vi "readFromTXTForXMLFiles.vi"(0 "input_path_dataSource":path, 5 "input_array_startTime":string[](array[string])=["1", "2"], 9 "input_array_endTime":string[](array[string])=["2", "3"]) -> (1 "paddle_TDD22":string[](array[string]), 2 "show_Terminal Point":dbl[](array[numeric]), 3 "show_array_TDD11":string[](array[string]), 4 "show_array_SDD21":string[](array[string]), 6 "show_array_SDD11_Max":string[](array[string]), 8 "show_array_ILD_Max":string[](array[string]), 10 "show_array_SCC11_Max":string[](array[string]), 11 "paddle_TDD11":string[](array[string]), 12 "show_array_Next":string[](array[string]), 13 "show_Cable Point":dbl[](array[numeric]), 14 "show_array_TDD22":string[](array[string]))   [LabVIEW 2011]
uses:
  <vilib>/Utility/file.llb/Read From Spreadsheet File (string).vi
panel:
  out "子数组":string[](array[string])
  out "show_array_index":dbl[](array[numeric])
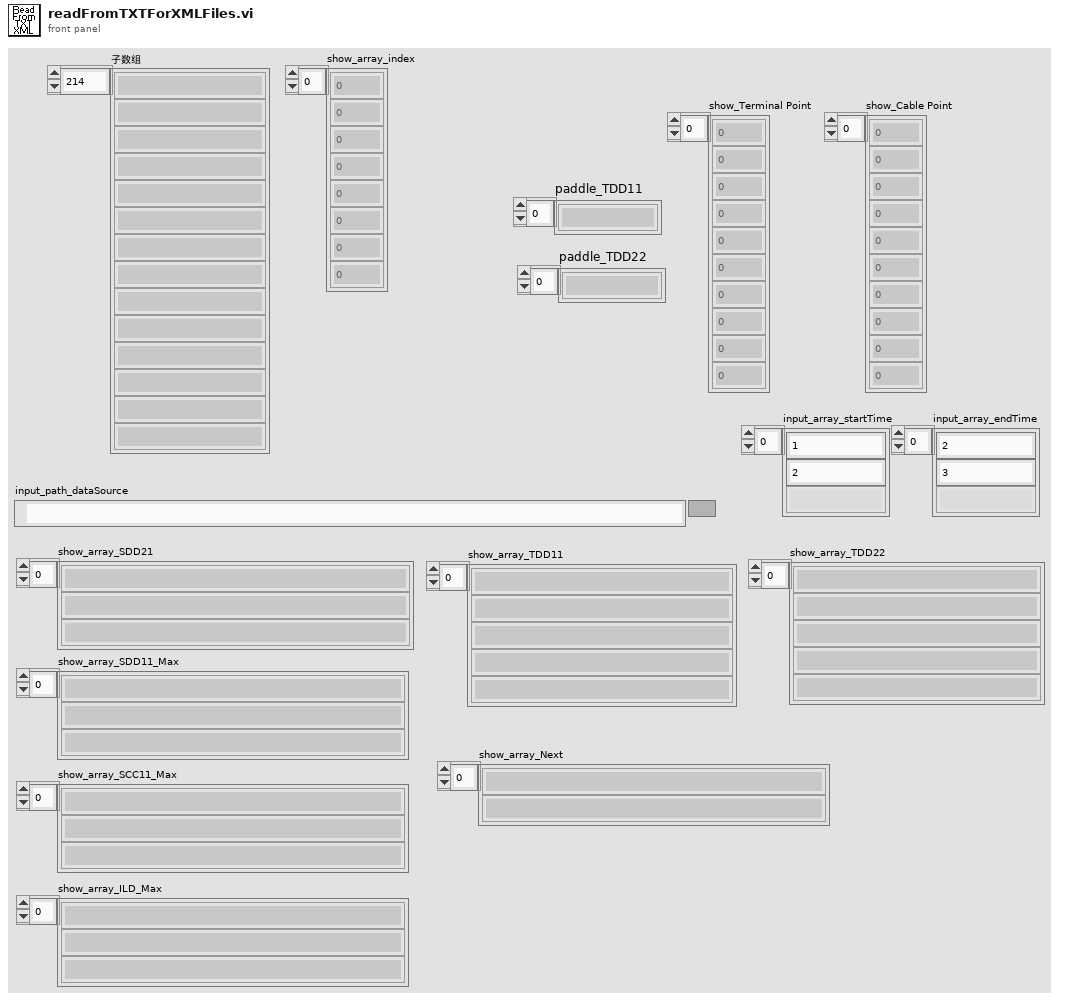
[diagram p1: front panel]
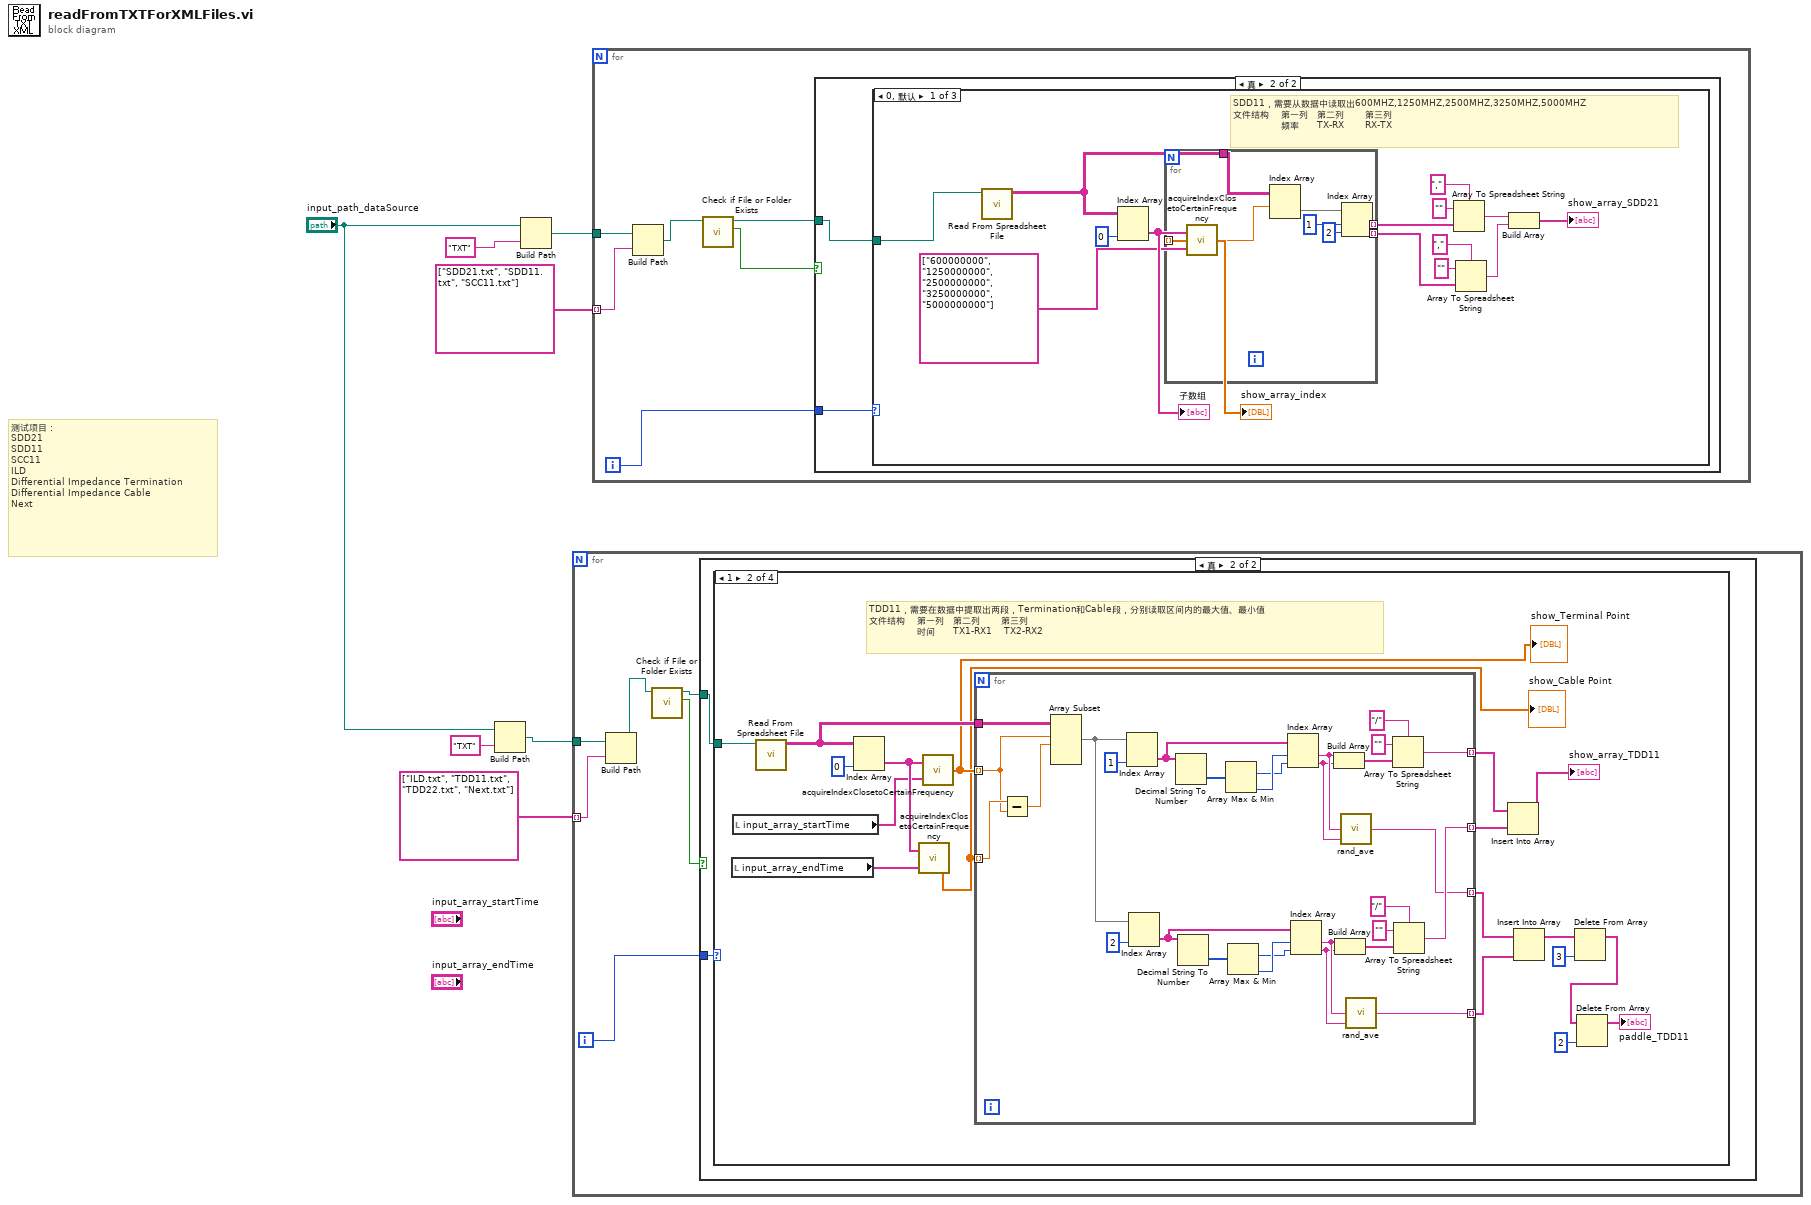
[diagram p0: block diagram]
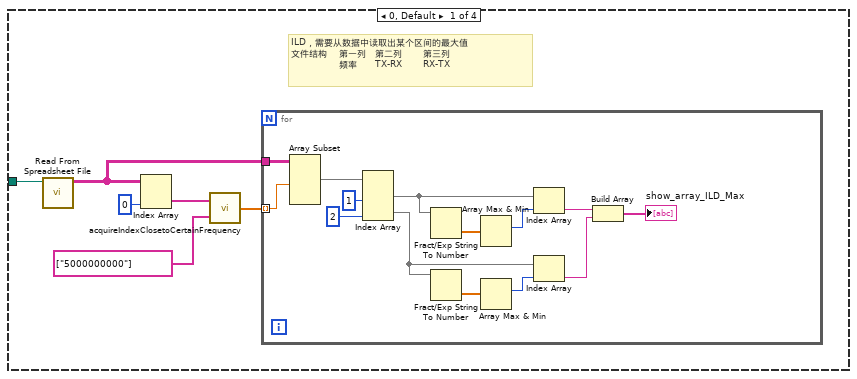
[diagram p3: hidden frame]
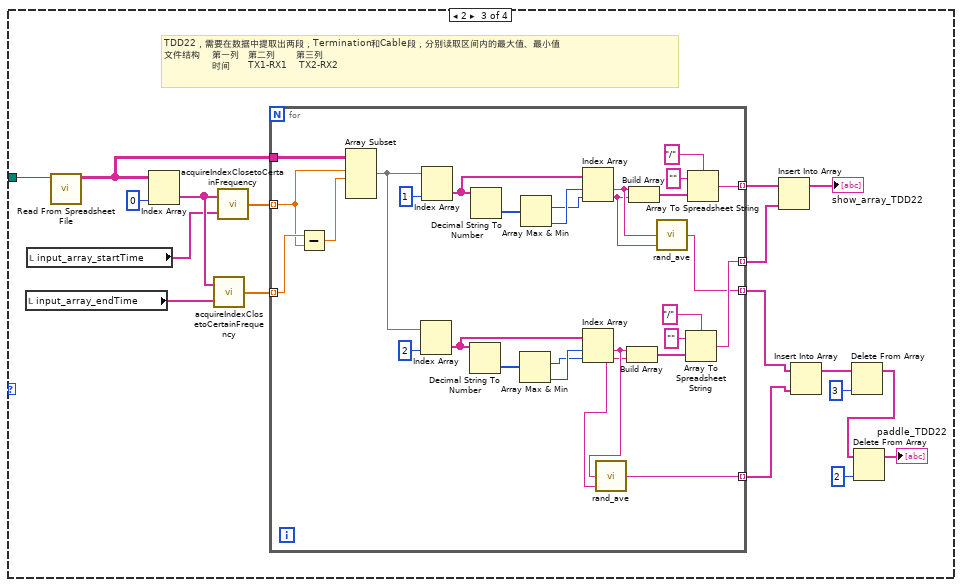
[diagram p4: hidden frame]
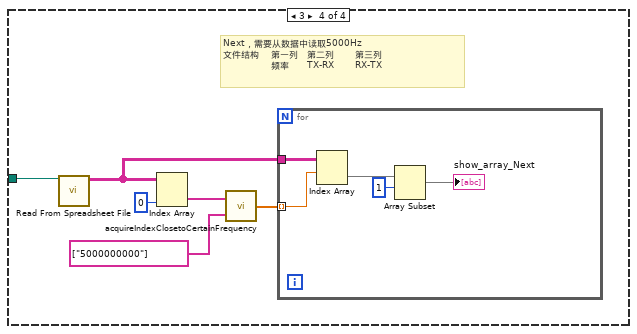
[diagram p5: hidden frame]
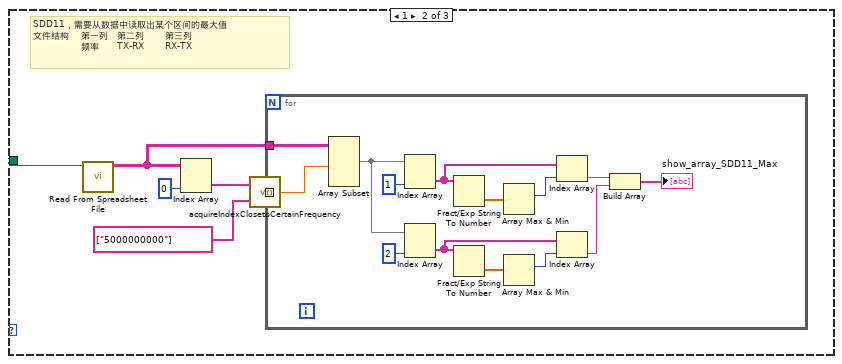
[diagram p7: hidden frame]
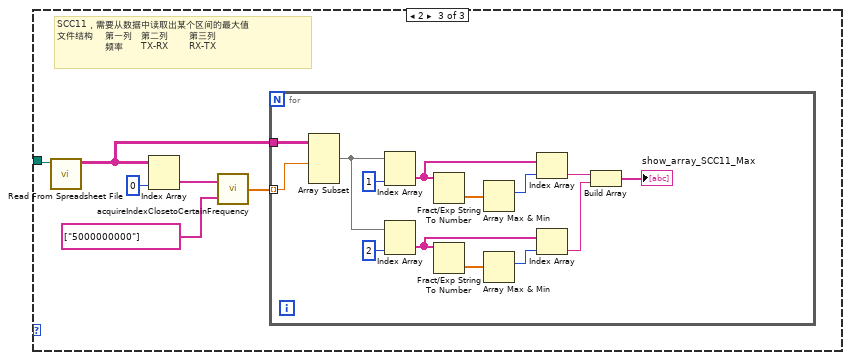
[diagram p8: hidden frame]
diagram:
  # "测试项目：\nSDD21\nSDD11\nSCC11\nILD\nDifferential Impedance Termination\nDifferential Impedance Cable\nNext"
  n1 = Build Path(base path="input_path_dataSource", name or relative path="TXT" ("名称或相对路径")) -> (appended path=w1:path)
  n2 = Build Path(base path="input_path_dataSource", name or relative path="TXT" ("名称或相对路径")) -> (appended path=w4:path)
  n3 = for {
    tunnel: string[] ["ILD.txt", "TDD11.txt", "TDD22.txt", "Next.txt"] -> [w12] mode=indexing
    tunnel: w1 -> [w13]
    i -> [w11]
    n4 = Build Path(base path=w13, name or relative path=w12) -> (appended path=w10:path)
    n5 = call <vilib>:"Check if File or Folder Exists.vi"("path"=w10) -> ("file or folder exists?"=w9:bool, "dup path"=w8:path)  [unwired: 8 in, 1 out]
    n6 = case shown="真" w9 {
      tunnel: w11 -> [_ w15]
      tunnel: w8 -> [_ w14]
      frame False {
      }
      frame True {
        n7 = case shown="1" w15 {
          tunnel: w14 -> [w21 w36 w97 w130]
          frame 0, Default {
            # "ILD，需要从数据中读取出某个区间的最大值\n文件结构    第一列   第二列       第三列       \n                频率      TX-RX       RX-TX"
            n8 = call-poly <vilib>:"Read From Spreadsheet File.vi"("file path (dialog if empty)"=w21) -> ("all rows"=w17:string[][])  [unwired: 6 in, 4 out]
            n9 = Index Array(array=w17, index (col)=0 ("禁用的索引 (列)")) -> (element=w19:string[])  [unwired: 1 in]
            n10 = call "acquireIndexClosetoCertainFrequency.vi"("input_array_freDemand"=string[] ["5000000000"], "input_array_freArray"=w19) -> ("show_array_index"=w16:dbl[])
            n11 = for {
              tunnel: w17 -> [w35]
              tunnel: w16 -> [w34] mode=indexing
              n12 = Array Subset(array=w35, length (row)=w34) -> (w33:string[][])  [unwired: 3 in]
              n13 = Index Array(array=w33, index (col) #1=1 ("禁用的索引 (列)"), index (col) #2=2 ("索引 (列)")) -> (element #1=w26:string[], element #2=w25:string[])  [unwired: 2 in]
              n14 = Fract/Exp String To Number(string=w26) -> (number=w30:dbl[])  [unwired: 3 in, 1 out]
              n15 = Fract/Exp String To Number(string=w25) -> (number=w29:dbl[])  [unwired: 3 in, 1 out]
              n16 = Array Max & Min(array=w30) -> (max index (indices)=w28:i32)  [unwired: 3 out]
              n17 = Array Max & Min(array=w29) -> (max index (indices)=w27:i32)  [unwired: 3 out]
              n18 = Index Array(array=w26, index=w28) -> (element=w23:string)
              n19 = Index Array(array=w25, index=w27) -> (element=w22:string)
              n20 = Build Array(w23, w22) -> (→"show_array_ILD_Max":string[])
            }
          }
          frame 1 {
            # "TDD11，需要在数据中提取出两段，Termination和Cable段，分别读取区间内的最大值、最小值\n文件结构    第一列   第二列       第三列\n                时间      TX1-RX1    TX2-RX2"
            n21 = local read "input_array_endTime"() -> (w45:string[])
            n22 = local read "input_array_startTime"() -> (w44:string[])
            n23 = call-poly <vilib>:"Read From Spreadsheet File.vi"("file path (dialog if empty)"=w36) -> ("all rows"=w52:string[][])  [unwired: 6 in, 4 out]
            n24 = Index Array(array=w52, index (col)=0 ("禁用的索引 (列)")) -> (element=w50:string[])  [unwired: 1 in]
            n25 = call "acquireIndexClosetoCertainFrequency.vi"("input_array_freDemand"=w45, "input_array_freArray"=w50) -> ("show_array_index"=w49:dbl[])
            "show_Cable Point" <- w49
            n26 = call "acquireIndexClosetoCertainFrequency.vi"("input_array_freDemand"=w44, "input_array_freArray"=w50) -> ("show_array_index"=w51:dbl[])
            "show_Terminal Point" <- w51
            n27 = for {
              tunnel: w52 -> [w82]
              tunnel: w51 -> [w73] mode=indexing
              tunnel: w49 -> [w74] mode=indexing
              tunnel: [w65] -> w48 mode=indexing
              tunnel: [w64] -> w47 mode=indexing
              tunnel: [w55] -> w38 mode=indexing
              tunnel: [w54] -> w37 mode=indexing
              n28 = Subtract(x=w74, y=w73) -> (x-y=w72:dbl)
              n29 = Array Subset(array=w82, index (row)=w73, length (row)=w72) -> (w79:string[][])  [unwired: 2 in]
              n30 = Index Array(array=w79, index (col)=1 ("禁用的索引 (列)")) -> (element=w76:string[])  [unwired: 1 in]
              n31 = Index Array(array=w79, index (col)=2 ("禁用的索引 (列)")) -> (element=w75:string[])  [unwired: 1 in]
              n32 = Decimal String To Number(string=w76) -> (number=w78:i32[])  [unwired: 2 in, 1 out]
              n33 = Decimal String To Number(string=w75) -> (number=w77:i32[])  [unwired: 2 in, 1 out]
              n34 = Array Max & Min(array=w78) -> (max index (indices)=w62:i32, min index (indices)=w63:i32)  [unwired: 2 out]
              n35 = Array Max & Min(array=w77) -> (max index (indices)=w60:i32, min index (indices)=w61:i32)  [unwired: 2 out]
              n36 = Index Array(array=w76, index #1=w63, index #2=w62) -> (element #1=w59:string, element #2=w58:string)
              n37 = Index Array(array=w75, index #1=w61, index #2=w60) -> (element #1=w57:string, element #2=w56:string)
              n38 = Build Array(w59, w58) -> (w69:string[])
              n39 = Build Array(w57, w56) -> (w68:string[])
              n40 = call "rand_ave.vi"("最小值"=w58, "最大值"=w59) -> ("结果"=w54:string)  [unwired: 1 in]
              n41 = call "rand_ave.vi"("最小值"=w56, "最大值"=w57) -> ("结果"=w55:string)  [unwired: 1 in]
              n42 = Array To Spreadsheet String(delimiter (Tab)="/" ("分隔符(Tab)"), array=w69, 3:"" ("格式字符串")) -> (spreadsheet string=w65:string)
              n43 = Array To Spreadsheet String(delimiter (Tab)="/" ("分隔符(Tab)"), array=w68, 3:"" ("格式字符串")) -> (spreadsheet string=w64:string)
            }
            n44 = Insert Into Array(array=w48, new element=w47) -> (→"show_array_TDD11":string[])  [unwired: 1 in]
            n45 = Insert Into Array(array=w37, new element=w38) -> (w43:string[])  [unwired: 1 in]
            n46 = Delete From Array(array=w43, index=3 ("索引")) -> (array with subset deleted=w41:string[])  [unwired: 1 in, 1 out]
            n47 = Delete From Array(array=w41, index=2 ("索引")) -> (array with subset deleted=→"paddle_TDD11":string[])  [unwired: 1 in, 1 out]
          }
          frame 2 {
            # "TDD22，需要在数据中提取出两段，Termination和Cable段，分别读取区间内的最大值、最小值\n文件结构    第一列   第二列       第三列\n                时间      TX1-RX1    TX2-RX2"
            n48 = local read "input_array_endTime"() -> (w90:string[])
            n49 = local read "input_array_startTime"() -> (w91:string[])
            n50 = call-poly <vilib>:"Read From Spreadsheet File.vi"("file path (dialog if empty)"=w97) -> ("all rows"=w99:string[][])  [unwired: 6 in, 4 out]
            n51 = Index Array(array=w99, index (col)=0 ("禁用的索引 (列)")) -> (element=w96:string[])  [unwired: 1 in]
            n52 = call "acquireIndexClosetoCertainFrequency.vi"("input_array_freDemand"=w90, "input_array_freArray"=w96) -> ("show_array_index"=w95:dbl[])
            n53 = call "acquireIndexClosetoCertainFrequency.vi"("input_array_freDemand"=w91, "input_array_freArray"=w96) -> ("show_array_index"=w98:dbl[])
            n54 = for {
              tunnel: w99 -> [w129]
              tunnel: w98 -> [w120] mode=indexing
              tunnel: w95 -> [w121] mode=indexing
              tunnel: [w112] -> w94 mode=indexing
              tunnel: [w111] -> w93 mode=indexing
              tunnel: [w103] -> w89 mode=indexing
              tunnel: [w106] -> w88 mode=indexing
              n55 = Subtract(x=w121, y=w120) -> (x-y=w119:dbl)
              n56 = Array Subset(array=w129, index (row)=w120, length (row)=w119) -> (w126:string[][])  [unwired: 2 in]
              n57 = Index Array(array=w126, index (col)=2 ("禁用的索引 (列)")) -> (element=w122:string[])  [unwired: 1 in]
              n58 = Index Array(array=w126, index (col)=1 ("禁用的索引 (列)")) -> (element=w123:string[])  [unwired: 1 in]
              n59 = Decimal String To Number(string=w122) -> (number=w124:i32[])  [unwired: 2 in, 1 out]
              n60 = Decimal String To Number(string=w123) -> (number=w125:i32[])  [unwired: 2 in, 1 out]
              n61 = Array Max & Min(array=w124) -> (max index (indices)=w107:i32, min index (indices)=w108:i32)  [unwired: 2 out]
              n62 = Array Max & Min(array=w125) -> (max index (indices)=w109:i32, min index (indices)=w110:i32)  [unwired: 2 out]
              n63 = Index Array(array=w123, index #1=w110, index #2=w109) -> (element #1=w105:string, element #2=w104:string)
              n64 = Index Array(array=w122, index #1=w108, index #2=w107) -> (element #1=w102:string, element #2=w101:string)
              n65 = call "rand_ave.vi"("最小值"=w101, "最大值"=w102) -> ("结果"=w106:string)  [unwired: 1 in]
              n66 = Build Array(w102, w101) -> (w115:string[])
              n67 = Build Array(w105, w104) -> (w116:string[])
              n68 = call "rand_ave.vi"("最小值"=w104, "最大值"=w105) -> ("结果"=w103:string)  [unwired: 1 in]
              n69 = Array To Spreadsheet String(delimiter (Tab)="/" ("分隔符(Tab)"), array=w115, 3:"" ("格式字符串")) -> (spreadsheet string=w111:string)
              n70 = Array To Spreadsheet String(delimiter (Tab)="/" ("分隔符(Tab)"), array=w116, 3:"" ("格式字符串")) -> (spreadsheet string=w112:string)
            }
            n71 = Insert Into Array(array=w94, new element=w93) -> (→"show_array_TDD22":string[])  [unwired: 1 in]
            n72 = Insert Into Array(array=w89, new element=w88) -> (w87:string[])  [unwired: 1 in]
            n73 = Delete From Array(array=w87, index=3 ("索引")) -> (array with subset deleted=w85:string[])  [unwired: 1 in, 1 out]
            n74 = Delete From Array(array=w85, index=2 ("索引")) -> (array with subset deleted=→"paddle_TDD22":string[])  [unwired: 1 in, 1 out]
          }
          frame 3 {
            # "Next，需要从数据中读取5000Hz\n文件结构    第一列   第二列       第三列       \n                频率      TX-RX       RX-TX"
            n75 = call-poly <vilib>:"Read From Spreadsheet File.vi"("file path (dialog if empty)"=w130) -> ("all rows"=w134:string[][])  [unwired: 6 in, 4 out]
            n76 = Index Array(array=w134, index (col)=0 ("禁用的索引 (列)")) -> (element=w132:string[])  [unwired: 1 in]
            n77 = call "acquireIndexClosetoCertainFrequency.vi"("input_array_freDemand"=string[] ["5000000000"], "input_array_freArray"=w132) -> ("show_array_index"=w135:dbl[])
            n78 = for {
              tunnel: w134 -> [w140]
              tunnel: w135 -> [w136] mode=indexing
              n79 = Index Array(array=w140, index (row)=w136) -> (element=w139:string[])  [unwired: 1 in]
              n80 = Array Subset(array=w139, index=1 ("索引")) -> (→"show_array_Next":string[])  [unwired: 1 in]
            }
          }
        }
      }
    }
  }
  n81 = for {
    tunnel: string[] ["SDD21.txt", "SDD11.txt", "SCC11.txt"] -> [w145] mode=indexing
    tunnel: w4 -> [w146]
    i -> [w144]
    n82 = Build Path(base path=w146, name or relative path=w145) -> (appended path=w143:path)
    n83 = call <vilib>:"Check if File or Folder Exists.vi"("path"=w143) -> ("file or folder exists?"=w142:bool, "dup path"=w141:path)  [unwired: 8 in, 1 out]
    n84 = case shown="真" w142 {
      tunnel: w144 -> [_ w148]
      tunnel: w141 -> [_ w147]
      frame False {
      }
      frame True {
        n85 = case shown="0, 默认" w148 {
          tunnel: w147 -> [w163 w171 w191]
          frame 0, Default {
            # "SDD11，需要从数据中读取出600MHZ,1250MHZ,2500MHZ,3250MHZ,5000MHZ\n文件结构    第一列   第二列       第三列       \n                频率      TX-RX       RX-TX"
            n86 = call-poly <vilib>:"Read From Spreadsheet File.vi"("file path (dialog if empty)"=w163) -> ("all rows"=w159:string[][])  [unwired: 6 in, 4 out]
            n87 = Index Array(array=w159, index (col)=0 ("禁用的索引 (列)")) -> (element=w161:string[])  [unwired: 1 in]
            "子数组" <- w161
            n88 = call "acquireIndexClosetoCertainFrequency.vi"("input_array_freDemand"=string[] ["600000000", "1250000000", "2500000000", "3250000000", "5000000000"], "input_array_freArray"=w161) -> ("show_array_index"=w158:dbl[])
            "show_array_index" <- w158
            n89 = for {
              tunnel: w159 -> [w170]
              tunnel: w158 -> [w169] mode=indexing
              tunnel: [w165] -> w155 mode=indexing
              tunnel: [w164] -> w152 mode=indexing
              n90 = Index Array(array=w170, index (row)=w169) -> (element=w168:string[])  [unwired: 1 in]
              n91 = Index Array(array=w168, index #1=1 ("索引"), index #2=2 ("索引")) -> (element #1=w165:string, element #2=w164:string)
            }
            n92 = Array To Spreadsheet String(delimiter (Tab)="," ("分隔符(Tab)"), array=w155, 3:"" ("格式字符串")) -> (spreadsheet string=w151:string)
            n93 = Array To Spreadsheet String(delimiter (Tab)="," ("分隔符(Tab)"), array=w152, 3:"" ("格式字符串")) -> (spreadsheet string=w150:string)
            n94 = Build Array(w151, w150) -> (→"show_array_SDD21":string[])
          }
          frame 1 {
            # "SDD11，需要从数据中读取出某个区间的最大值\n文件结构    第一列   第二列       第三列       \n                频率      TX-RX       RX-TX"
            n95 = call-poly <vilib>:"Read From Spreadsheet File.vi"("file path (dialog if empty)"=w171) -> ("all rows"=w173:string[][])  [unwired: 6 in, 4 out]
            n96 = Index Array(array=w173, index (col)=0 ("禁用的索引 (列)")) -> (element=w175:string[])  [unwired: 1 in]
            n97 = call "acquireIndexClosetoCertainFrequency.vi"("input_array_freDemand"=string[] ["5000000000"], "input_array_freArray"=w175) -> ("show_array_index"=w172:dbl[])
            n98 = for {
              tunnel: w173 -> [w190]
              tunnel: w172 -> [w189] mode=indexing
              n99 = Array Subset(array=w190, length (row)=w189) -> (w186:string[][])  [unwired: 3 in]
              n100 = Index Array(array=w186, index (col)=1 ("禁用的索引 (列)")) -> (element=w183:string[])  [unwired: 1 in]
              n101 = Index Array(array=w186, index (col)=2 ("禁用的索引 (列)")) -> (element=w180:string[])  [unwired: 1 in]
              n102 = Fract/Exp String To Number(string=w183) -> (number=w185:dbl[])  [unwired: 3 in, 1 out]
              n103 = Fract/Exp String To Number(string=w180) -> (number=w184:dbl[])  [unwired: 3 in, 1 out]
              n104 = Array Max & Min(array=w185) -> (max index (indices)=w182:i32)  [unwired: 3 out]
              n105 = Array Max & Min(array=w184) -> (max index (indices)=w181:i32)  [unwired: 3 out]
              n106 = Index Array(array=w183, index=w182) -> (element=w179:string)
              n107 = Index Array(array=w180, index=w181) -> (element=w178:string)
              n108 = Build Array(w179, w178) -> (→"show_array_SDD11_Max":string[])
            }
          }
          frame 2 {
            # "SCC11，需要从数据中读取出某个区间的最大值\n文件结构    第一列   第二列       第三列       \n                频率      TX-RX       RX-TX"
            n109 = call-poly <vilib>:"Read From Spreadsheet File.vi"("file path (dialog if empty)"=w191) -> ("all rows"=w193:string[][])  [unwired: 6 in, 4 out]
            n110 = Index Array(array=w193, index (col)=0 ("禁用的索引 (列)")) -> (element=w195:string[])  [unwired: 1 in]
            n111 = call "acquireIndexClosetoCertainFrequency.vi"("input_array_freDemand"=string[] ["5000000000"], "input_array_freArray"=w195) -> ("show_array_index"=w192:dbl[])
            n112 = for {
              tunnel: w193 -> [w210]
              tunnel: w192 -> [w209] mode=indexing
              n113 = Array Subset(array=w210, length (row)=w209) -> (w206:string[][])  [unwired: 3 in]
              n114 = Index Array(array=w206, index (col)=1 ("禁用的索引 (列)")) -> (element=w203:string[])  [unwired: 1 in]
              n115 = Index Array(array=w206, index (col)=2 ("禁用的索引 (列)")) -> (element=w200:string[])  [unwired: 1 in]
              n116 = Fract/Exp String To Number(string=w203) -> (number=w205:dbl[])  [unwired: 3 in, 1 out]
              n117 = Fract/Exp String To Number(string=w200) -> (number=w204:dbl[])  [unwired: 3 in, 1 out]
              n118 = Array Max & Min(array=w205) -> (max index (indices)=w202:i32)  [unwired: 3 out]
              n119 = Array Max & Min(array=w204) -> (max index (indices)=w201:i32)  [unwired: 3 out]
              n120 = Index Array(array=w203, index=w202) -> (element=w199:string)
              n121 = Index Array(array=w200, index=w201) -> (element=w198:string)
              n122 = Build Array(w199, w198) -> (→"show_array_SCC11_Max":string[])
            }
          }
        }
      }
    }
  }
